vi "niSwitch Relay Control Wrapper.vi"(8 "error in":errorcluster, 9 "relay action (Close Relay)":T1=21 items=["Open Relay"=20, "Close Relay"=21], 10 "relay names":string, 11 "session factory in":refnum<class "Session Factory.lvclass">) -> (0 "error out":errorcluster, 3 "session factory out":refnum<class "Session Factory.lvclass">)   [LabVIEW 2021, in "Session Management niSwitch.lvlib" / "Session Factory.lvclass"]
doc: "Controls individual relays of the switch module. When controlling individual relays, the protection offered by setting the usage of source channels and configurations channels is void."
uses:
  Session Factory.lvclass
  <instrlib>/niSwitch/niSwitch.llb/niSwitch Relay Action.ctl
  NI Switch Client/RPC Messages/niswitch_grpc_RelayControlRequest.ctl
  NI Switch Client/RPC Messages/nidevice_grpc_Session.ctl
  NI Switch Client/RPC Messages/nidevice_grpc_Session_session/nidevice_grpc_Session_session.lvclass
  NI Switch Client/RPC Messages/niswitch_grpc_RelayControlRequest_relay_action_enum/niswitch_grpc_RelayControlRequest_relay_action_enum.lvclass
  Session Factory.lvclass/Session Factory.ctl
  NI Switch Client/RPC Messages/niswitch_grpc_RelayAction.ctl
  NI Switch Client/RPC Messages/niswitch_grpc_RelayControlRequest_relay_action_enum/niswitch_grpc_RelayControlRequest_relay_action_enum.lvclass/niswitch_grpc_RelayControlRequest_relay_action_enum.ctl
  NI Switch Client/NI Switch Client.lvlib
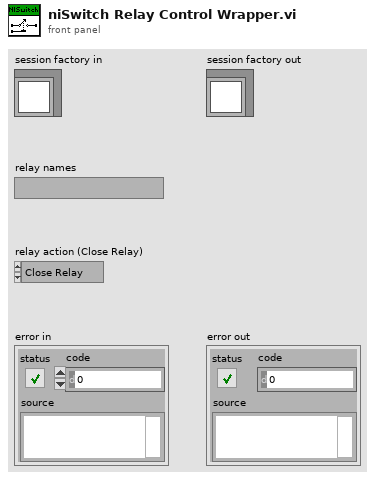
[diagram p1: front panel]
types:
  T1 = typedef "niSwitch Relay Action.ctl" = i32
  T2 = typedef "NI Switch Client.lvlib/niswitch_grpc_RelayControlRequest.ctl" = cluster{"vi":T3, "relay_name":string, "niswitch_grpc_RelayControlRequest_relay_action_enum":refnum<class "niswitch_grpc_RelayControlRequest_relay_action_enum.lvclass">}
  T3 = typedef "NI Switch Client.lvlib/nidevice_grpc_Session.ctl" = cluster{"nidevice_grpc_Session_session":refnum<class "nidevice_grpc_Session_session.lvclass">}
  T4 = typedef "NI Switch Client.lvlib/niswitch_grpc_RelayAction.ctl" = enum32{"RELAY_ACTION_UNSPECIFIED", "RELAY_ACTION_NISWITCH_VAL_OPEN_RELAY", "RELAY_ACTION_NISWITCH_VAL_CLOSE_RELAY"}
  T5 = typedef "grpc-lvsupport-release.lvlib/grpcId.ctl" = u64
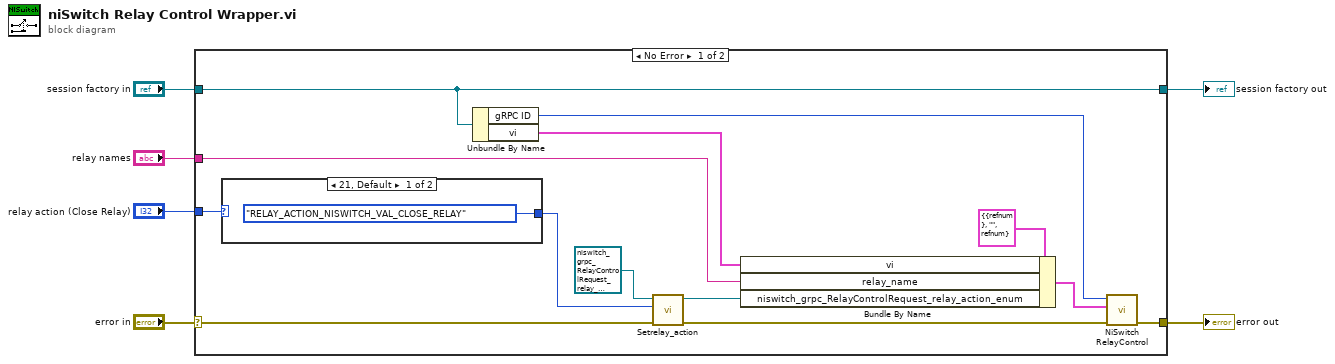
[diagram p0: block diagram]
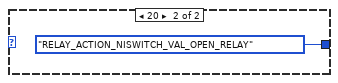
[diagram p2: hidden frame]
diagram:
  n1 = case shown="No Error" "error in" {
    selector: "error in" -> [w19 w22]
    tunnel: [w8 w23] -> w6
    tunnel: "session factory in" -> [w8 w23]
    tunnel: "relay names" -> [w12 _]
    tunnel: "relay action (Close Relay)" -> [w10 _]
    tunnel: [w9 w22] -> w5
    frame No Error {
      n2 = case shown="21, Default" w10 {
        tunnel: [niswitch_grpc_RelayAction."RELAY_ACTION_NISWITCH_VAL_CLOSE_RELAY" ("Set_Val") niswitch_grpc_RelayAction."RELAY_ACTION_NISWITCH_VAL_OPEN_RELAY" ("Set_Val")] -> w13
        frame 21, Default {
        }
        frame 20 {
        }
      }
      n3 = Unbundle By Name(w8) -> ("gRPC ID"=w16:T5, "vi"=w14:T3)
      n4 = call "Setrelay_action.vi"("error in (no error)"=w19, "Set_Val"=w13, "OneOfTemplate in"=refnum<class "niswitch_grpc_RelayControlRequest_relay_action_enum.lvclass"> refnum) -> ("error out"=w17:errorcluster, "OneOfTemplate out"=w7:refnum<class "niswitch_grpc_RelayControlRequest_relay_action_enum.lvclass">)  [unwired: 7 in]
      n5 = Bundle By Name(cluster=T2 {"vi"={"nidevice_grpc_Session_session"=refnum}, "relay_name"="", "niswitch_grpc_RelayControlRequest_relay_action_enum"=refnum} ("Request Data"), "vi"=w14, "relay_name"=w12, "niswitch_grpc_RelayControlRequest_relay_action_enum"=w7) -> (w15:T2)
      n6 = call "NiSwitch RelayControl.vi"("error in"=w17, "Request Data"=w15, "gRPC ID"=w16) -> ("error out"=w9:errorcluster)  [unwired: 6 in, 2 out]
    }
    frame Error {
    }
  }
  "error out" <- w5
  "session factory out" <- w6
